vi "Test Read-Write Control Text.vi"(8 "error in (no error)":errorcluster) -> (0 "error out":errorcluster, 3 "Pass?":bool)   [LabVIEW 2020]
uses:
  G-Unicode/Types/UTF-8 String/UTF-8 String.lvclass/UTF-8 String.ctl
  G-Unicode/Dialog & User Interface/Polymorphic VIs/Write Control Text/Write Listbox Header (UTF-8 String).vi
  G-Unicode/Dialog & User Interface/Polymorphic VIs/Read Control Text/Read Listbox Header (UTF-8 String).vi
  47e1521e-4900-4e50-93d0-971907de44b7.vi
  G-Unicode/Dialog & User Interface/Polymorphic VIs/Write Control Text/Write Graph Plot Names (UTF-8 String).vi
  G-Unicode/Dialog & User Interface/Polymorphic VIs/Write Control Text/Write Graph Cursor Names (UTF-8 String).vi
  G-Unicode/Dialog & User Interface/Polymorphic VIs/Write Control Text/Write Graph Axis Labels (UTF-8 String).vi
  G-Unicode/Dialog & User Interface/Polymorphic VIs/Write Control Text/Write Table Headers (UTF-8 String).vi
  G-Unicode/Dialog & User Interface/Polymorphic VIs/Read Control Text/Read Table Headers (UTF-8 String).vi
  cbd299b7-ed5c-44d8-98e3-4b07b256a3af.vi
  97e6e9dd-fb41-465e-8130-768105b8566a.vi
  G-Unicode/Dialog & User Interface/Polymorphic VIs/Write Control Text/Write Multicolumn Listbox Headers (UTF-8 String).vi
  G-Unicode/Dialog & User Interface/Polymorphic VIs/Read Control Text/Read Multicolumn Listbox Headers (UTF-8 String).vi
  2cb1db3a-9545-49da-8e46-b28431192bfb.vi
  d3ca7cbe-fe55-4c08-9226-8df1279bea32.vi
  G-Unicode/Dialog & User Interface/Polymorphic VIs/Write Control Text/Write Radio Button Text (UTF-8 String).vi
  G-Unicode/Dialog & User Interface/Polymorphic VIs/Read Control Text/Read Radio Button Text (UTF-8 String).vi
  c66c8a8e-6384-46dd-ad34-c6b36e981c5f.vi
  G-Unicode/Dialog & User Interface/Polymorphic VIs/Write Control Text/Write Tab Pages (UTF-8 String).vi
  G-Unicode/Dialog & User Interface/Polymorphic VIs/Read Control Text/Read Tab Pages (UTF-8 String).vi
  11ce0e2c-e1a8-46a3-af78-7df26efc8245.vi
  G-Unicode/Dialog & User Interface/Polymorphic VIs/Write Control Text/Write Listbox Items (UTF-8 String).vi
  G-Unicode/Dialog & User Interface/Polymorphic VIs/Read Control Text/Read Listbox Items (UTF-8 String).vi
  c5b5f753-7993-4590-ab7a-38cd070e680f.vi
  G-Unicode/Dialog & User Interface/Polymorphic VIs/Write Control Text/Write Table Value (UTF-8 String).vi
  G-Unicode/Dialog & User Interface/Polymorphic VIs/Read Control Text/Read Table Value (UTF-8 String).vi
  d87d6912-68ee-4c4f-8e1f-9eaf2c3e8737.vi
  G-Unicode/Dialog & User Interface/Polymorphic VIs/Write Control Text/Write Ring Strings (UTF-8 String).vi
  G-Unicode/Dialog & User Interface/Polymorphic VIs/Read Control Text/Read Ring Strings (UTF-8 String).vi
  b51df372-b908-46a9-9cd9-1bce9bcba761.vi
  3f50c59c-438d-4159-8265-e7e5e4819d1d.vi
  G-Unicode/Dialog & User Interface/Polymorphic VIs/Write Control Text/Write 2D String Array Value (UTF-8 String).vi
  G-Unicode/Dialog & User Interface/Polymorphic VIs/Read Control Text/Read 2D String Array Value (UTF-8 String).vi
  f481c7ac-37a4-4879-9d59-93dd94c77838.vi
  G-Unicode/Dialog & User Interface/Polymorphic VIs/Write Control Text/Write 1D String Array Value (UTF-8 String).vi
  G-Unicode/Dialog & User Interface/Polymorphic VIs/Read Control Text/Read 1D String Array Value (UTF-8 String).vi
  2abff34c-ba54-40bb-bfb0-e7a9eb1a66c8.vi
  G-Unicode/Dialog & User Interface/Polymorphic VIs/Write Control Text/Write String Value (UTF-8 String).vi
  G-Unicode/Dialog & User Interface/Polymorphic VIs/Read Control Text/Read String Value (UTF-8 String).vi
  b9bba32d-5ca2-4258-b841-0da24b58b874.vi
  G-Unicode/Dialog & User Interface/Polymorphic VIs/Write Control Text/Write Multicolumn Listbox Items (UTF-8 String).vi
  G-Unicode/Dialog & User Interface/Polymorphic VIs/Read Control Text/Read Multicolumn Listbox Items (UTF-8 String).vi
  4c20338b-6e60-4a75-91ad-9e96f58f92b0.vi
  G-Unicode/Dialog & User Interface/Polymorphic VIs/Write Control Text/Write Listbox Header (UTF-8 String).vi/5206cb6b-04fb-41f5-a37e-29c14f142303.vi
  G-Unicode/Dialog & User Interface/Polymorphic VIs/Read Control Text/Read Listbox Header (UTF-8 String).vi/bfba3187-b22e-4285-8cc2-1816a803f974.vi
  47e1521e-4900-4e50-93d0-971907de44b7.vi/3a31b270-3bb6-4c58-a256-c5fcc2c98f09.vi
  47e1521e-4900-4e50-93d0-971907de44b7.vi/0ec5df2d-ef9b-4f84-a6a8-ffcedd45c4dc.vi
  G-Unicode/Dialog & User Interface/Polymorphic VIs/Write Control Text/Write Graph Plot Names (UTF-8 String).vi/5206cb6b-04fb-41f5-a37e-29c14f142303.vi
  G-Unicode/Dialog & User Interface/Polymorphic VIs/Write Control Text/Write Graph Cursor Names (UTF-8 String).vi/5206cb6b-04fb-41f5-a37e-29c14f142303.vi
  G-Unicode/Dialog & User Interface/Polymorphic VIs/Write Control Text/Write Graph Axis Labels (UTF-8 String).vi/5206cb6b-04fb-41f5-a37e-29c14f142303.vi
  G-Unicode/Dialog & User Interface/Polymorphic VIs/Write Control Text/Write Graph Axis Labels (UTF-8 String).vi/dd8e371b-806c-4d03-8f90-d02a4c0388fb.vi
  G-Unicode/Dialog & User Interface/Polymorphic VIs/Write Control Text/Write Table Headers (UTF-8 String).vi/5206cb6b-04fb-41f5-a37e-29c14f142303.vi
  G-Unicode/Dialog & User Interface/Polymorphic VIs/Write Control Text/Write Table Headers (UTF-8 String).vi/ac01c1c3-6448-4046-bb74-48d1977bc508.vi
  G-Unicode/Dialog & User Interface/Polymorphic VIs/Read Control Text/Read Table Headers (UTF-8 String).vi/eedf47bc-7647-4a54-abe9-23d54898c809.vi
  G-Unicode/Dialog & User Interface/Polymorphic VIs/Read Control Text/Read Table Headers (UTF-8 String).vi/0d5c28b1-d47f-4710-9fb4-2778fb7e7b81.vi
  cbd299b7-ed5c-44d8-98e3-4b07b256a3af.vi/3a31b270-3bb6-4c58-a256-c5fcc2c98f09.vi
  cbd299b7-ed5c-44d8-98e3-4b07b256a3af.vi/0ec5df2d-ef9b-4f84-a6a8-ffcedd45c4dc.vi
  97e6e9dd-fb41-465e-8130-768105b8566a.vi/3a31b270-3bb6-4c58-a256-c5fcc2c98f09.vi
  97e6e9dd-fb41-465e-8130-768105b8566a.vi/0ec5df2d-ef9b-4f84-a6a8-ffcedd45c4dc.vi
  G-Unicode/Dialog & User Interface/Polymorphic VIs/Write Control Text/Write Multicolumn Listbox Headers (UTF-8 String).vi/5206cb6b-04fb-41f5-a37e-29c14f142303.vi
  G-Unicode/Dialog & User Interface/Polymorphic VIs/Write Control Text/Write Multicolumn Listbox Headers (UTF-8 String).vi/ac01c1c3-6448-4046-bb74-48d1977bc508.vi
  G-Unicode/Dialog & User Interface/Polymorphic VIs/Read Control Text/Read Multicolumn Listbox Headers (UTF-8 String).vi/f6f7f231-7ddf-476b-a943-0386d848a5c9.vi
  G-Unicode/Dialog & User Interface/Polymorphic VIs/Read Control Text/Read Multicolumn Listbox Headers (UTF-8 String).vi/fba5a6d2-cdfe-4afc-9e2c-d2641906be0d.vi
  2cb1db3a-9545-49da-8e46-b28431192bfb.vi/3a31b270-3bb6-4c58-a256-c5fcc2c98f09.vi
  2cb1db3a-9545-49da-8e46-b28431192bfb.vi/0ec5df2d-ef9b-4f84-a6a8-ffcedd45c4dc.vi
  d3ca7cbe-fe55-4c08-9226-8df1279bea32.vi/3a31b270-3bb6-4c58-a256-c5fcc2c98f09.vi
  d3ca7cbe-fe55-4c08-9226-8df1279bea32.vi/0ec5df2d-ef9b-4f84-a6a8-ffcedd45c4dc.vi
  G-Unicode/Dialog & User Interface/Polymorphic VIs/Write Control Text/Write Radio Button Text (UTF-8 String).vi/5206cb6b-04fb-41f5-a37e-29c14f142303.vi
  G-Unicode/Dialog & User Interface/Polymorphic VIs/Read Control Text/Read Radio Button Text (UTF-8 String).vi/f6f7f231-7ddf-476b-a943-0386d848a5c9.vi
  c66c8a8e-6384-46dd-ad34-c6b36e981c5f.vi/3a31b270-3bb6-4c58-a256-c5fcc2c98f09.vi
  c66c8a8e-6384-46dd-ad34-c6b36e981c5f.vi/0ec5df2d-ef9b-4f84-a6a8-ffcedd45c4dc.vi
  G-Unicode/Dialog & User Interface/Polymorphic VIs/Write Control Text/Write Tab Pages (UTF-8 String).vi/5206cb6b-04fb-41f5-a37e-29c14f142303.vi
  G-Unicode/Dialog & User Interface/Polymorphic VIs/Read Control Text/Read Tab Pages (UTF-8 String).vi/f6f7f231-7ddf-476b-a943-0386d848a5c9.vi
  11ce0e2c-e1a8-46a3-af78-7df26efc8245.vi/3a31b270-3bb6-4c58-a256-c5fcc2c98f09.vi
  11ce0e2c-e1a8-46a3-af78-7df26efc8245.vi/0ec5df2d-ef9b-4f84-a6a8-ffcedd45c4dc.vi
  G-Unicode/Dialog & User Interface/Polymorphic VIs/Write Control Text/Write Listbox Items (UTF-8 String).vi/5206cb6b-04fb-41f5-a37e-29c14f142303.vi
  G-Unicode/Dialog & User Interface/Polymorphic VIs/Read Control Text/Read Listbox Items (UTF-8 String).vi/f6f7f231-7ddf-476b-a943-0386d848a5c9.vi
  c5b5f753-7993-4590-ab7a-38cd070e680f.vi/3a31b270-3bb6-4c58-a256-c5fcc2c98f09.vi
  c5b5f753-7993-4590-ab7a-38cd070e680f.vi/0ec5df2d-ef9b-4f84-a6a8-ffcedd45c4dc.vi
  G-Unicode/Dialog & User Interface/Polymorphic VIs/Write Control Text/Write Table Value (UTF-8 String).vi/5206cb6b-04fb-41f5-a37e-29c14f142303.vi
  G-Unicode/Dialog & User Interface/Polymorphic VIs/Read Control Text/Read Table Value (UTF-8 String).vi/f6f7f231-7ddf-476b-a943-0386d848a5c9.vi
  d87d6912-68ee-4c4f-8e1f-9eaf2c3e8737.vi/3a31b270-3bb6-4c58-a256-c5fcc2c98f09.vi
  d87d6912-68ee-4c4f-8e1f-9eaf2c3e8737.vi/0ec5df2d-ef9b-4f84-a6a8-ffcedd45c4dc.vi
  G-Unicode/Dialog & User Interface/Polymorphic VIs/Write Control Text/Write Ring Strings (UTF-8 String).vi/5206cb6b-04fb-41f5-a37e-29c14f142303.vi
  G-Unicode/Dialog & User Interface/Polymorphic VIs/Read Control Text/Read Ring Strings (UTF-8 String).vi/f6f7f231-7ddf-476b-a943-0386d848a5c9.vi
  b51df372-b908-46a9-9cd9-1bce9bcba761.vi/3a31b270-3bb6-4c58-a256-c5fcc2c98f09.vi
  b51df372-b908-46a9-9cd9-1bce9bcba761.vi/0ec5df2d-ef9b-4f84-a6a8-ffcedd45c4dc.vi
  3f50c59c-438d-4159-8265-e7e5e4819d1d.vi/3a31b270-3bb6-4c58-a256-c5fcc2c98f09.vi
  3f50c59c-438d-4159-8265-e7e5e4819d1d.vi/0ec5df2d-ef9b-4f84-a6a8-ffcedd45c4dc.vi
  G-Unicode/Dialog & User Interface/Polymorphic VIs/Write Control Text/Write 2D String Array Value (UTF-8 String).vi/5206cb6b-04fb-41f5-a37e-29c14f142303.vi
  G-Unicode/Dialog & User Interface/Polymorphic VIs/Read Control Text/Read 2D String Array Value (UTF-8 String).vi/f6f7f231-7ddf-476b-a943-0386d848a5c9.vi
  f481c7ac-37a4-4879-9d59-93dd94c77838.vi/3a31b270-3bb6-4c58-a256-c5fcc2c98f09.vi
  f481c7ac-37a4-4879-9d59-93dd94c77838.vi/0ec5df2d-ef9b-4f84-a6a8-ffcedd45c4dc.vi
  G-Unicode/Dialog & User Interface/Polymorphic VIs/Write Control Text/Write 1D String Array Value (UTF-8 String).vi/5206cb6b-04fb-41f5-a37e-29c14f142303.vi
  G-Unicode/Dialog & User Interface/Polymorphic VIs/Read Control Text/Read 1D String Array Value (UTF-8 String).vi/f6f7f231-7ddf-476b-a943-0386d848a5c9.vi
  2abff34c-ba54-40bb-bfb0-e7a9eb1a66c8.vi/3a31b270-3bb6-4c58-a256-c5fcc2c98f09.vi
  2abff34c-ba54-40bb-bfb0-e7a9eb1a66c8.vi/0ec5df2d-ef9b-4f84-a6a8-ffcedd45c4dc.vi
  G-Unicode/Dialog & User Interface/Polymorphic VIs/Write Control Text/Write String Value (UTF-8 String).vi/5206cb6b-04fb-41f5-a37e-29c14f142303.vi
  G-Unicode/Dialog & User Interface/Polymorphic VIs/Read Control Text/Read String Value (UTF-8 String).vi/bfba3187-b22e-4285-8cc2-1816a803f974.vi
  b9bba32d-5ca2-4258-b841-0da24b58b874.vi/3a31b270-3bb6-4c58-a256-c5fcc2c98f09.vi
  b9bba32d-5ca2-4258-b841-0da24b58b874.vi/0ec5df2d-ef9b-4f84-a6a8-ffcedd45c4dc.vi
  G-Unicode/Dialog & User Interface/Polymorphic VIs/Write Control Text/Write Multicolumn Listbox Items (UTF-8 String).vi/5206cb6b-04fb-41f5-a37e-29c14f142303.vi
  G-Unicode/Dialog & User Interface/Polymorphic VIs/Read Control Text/Read Multicolumn Listbox Items (UTF-8 String).vi/f6f7f231-7ddf-476b-a943-0386d848a5c9.vi
  4c20338b-6e60-4a75-91ad-9e96f58f92b0.vi/3a31b270-3bb6-4c58-a256-c5fcc2c98f09.vi
  4c20338b-6e60-4a75-91ad-9e96f58f92b0.vi/0ec5df2d-ef9b-4f84-a6a8-ffcedd45c4dc.vi
  G-Unicode/Private/Conversion/Text as Encoded String.vi
  G-Unicode/Private/Conversion/Polymorphic VIs/Text as Encoded String (UTF-8 String).vi
  G-Unicode/Private/Conversion/Encoded UTF-8 String to Encoded UTF-16LE String.vi
  G-Unicode/Types/UTF-8 String/New UTF-8 String.vi
  G-Unicode/Types/UTF-8 String/Read Encoded UTF-8 String.vi
  G-Unicode/Unicode/Encode String.vi
  G-Unicode/Private/Conversion/Text to UTF-8.vi
  G-Unicode/Private/Conversion/Polymorphic VIs/Text to UTF-8 (LabVIEW String).vi
  G-Unicode/Unicode/SubVIs/UTF-16 Byte Swap.vi
  G-Unicode/Private/Conversion/UTF-8 to Text.vi
  G-Unicode/Private/Conversion/Polymorphic VIs/UTF-8 to Text (LabVIEW String).vi
  G-Unicode/Private/Conversion/Encoded UTF-16LE String to Encoded UTF-8 String.vi
  G-Unicode/Unicode/Prepend BOM.vi
  G-Unicode/Unicode/SubVIs/Byte Order Marks.vi
  G-Unicode/Unicode/Detect BOM.vi
  G-Unicode/Private/User Interface/Write String.vi
  G-Unicode/Private/User Interface/Read String.vi
  G-Unicode/Unicode/Detect String Encoding.vi
  G-Unicode/Private/User Interface/Write String Array (1D).vi
  G-Unicode/Private/User Interface/Read String Array (1D).vi
  G-Unicode/Private/User Interface/Write String Array (2D).vi
  G-Unicode/Private/User Interface/Read String Array (2D).vi
  G-Unicode/Private/User Interface/Write Ring Control.vi
  G-Unicode/Private/User Interface/Read Ring Control.vi
  G-Unicode/Private/User Interface/Write MultCol Listbox Data.vi
  G-Unicode/Private/User Interface/Read MultCol Listbox Data.vi
  G-Unicode/Private/User Interface/Write MultCol Listbox Headers.vi
  G-Unicode/Private/User Interface/Read MultCol Listbox Headers.vi
  G-Unicode/Private/User Interface/Write Listbox Data.vi
  G-Unicode/Private/User Interface/Read Listbox Data.vi
  G-Unicode/Private/User Interface/Write Listbox Header.vi
  G-Unicode/Private/User Interface/Read Listbox Header.vi
  G-Unicode/Private/User Interface/Write Table Data.vi
  G-Unicode/Private/User Interface/Read Table Data.vi
  G-Unicode/Private/User Interface/Write Table Headers.vi
  G-Unicode/Private/User Interface/Read Table Headers.vi
  G-Unicode/Private/User Interface/Write Tab Control.vi
  G-Unicode/Private/User Interface/Read Tab Control.vi
  G-Unicode/Private/User Interface/Write Radio Buttons.vi
  G-Unicode/Private/User Interface/Read Radio Button Text.vi
  G-Unicode/Private/User Interface/Write Graph-Chart Plot Names.vi
  G-Unicode/Private/User Interface/Write Graph-Chart Axis Labels.vi
  G-Unicode/Private/User Interface/Write Graph-Chart Cursor Names.vi
  G-Unicode/Types/UTF-8 String/UTF-8 String.lvclass
  G-Unicode/G-Unicode.lvlib
panel:
  out "Waveform Graph":dbl[](graph)
  out "Waveform Chart":dbl(graph)
  in  "Radio Buttons":T1(radio)
  in  "Tab Control":enum32{"Page 1", "Page 2", "Page 3", "Page 4"}(tab)
  in  "Multicolumn Listbox":i32(listbox)
  in  "Listbox":i32(listbox)
  in  "Table Control":string[][](table)
  in  "Menu Ring":u16(ring)
  in  "Text Ring":u16(ring)
  in  "String Array (2D)":string[][](array[string])
  in  "String Array (1D)":string[](array[string])
  in  "String":string
  # "Note the dropdowns for the ring controls aren't rendered correctly, but when selected it looks OK."
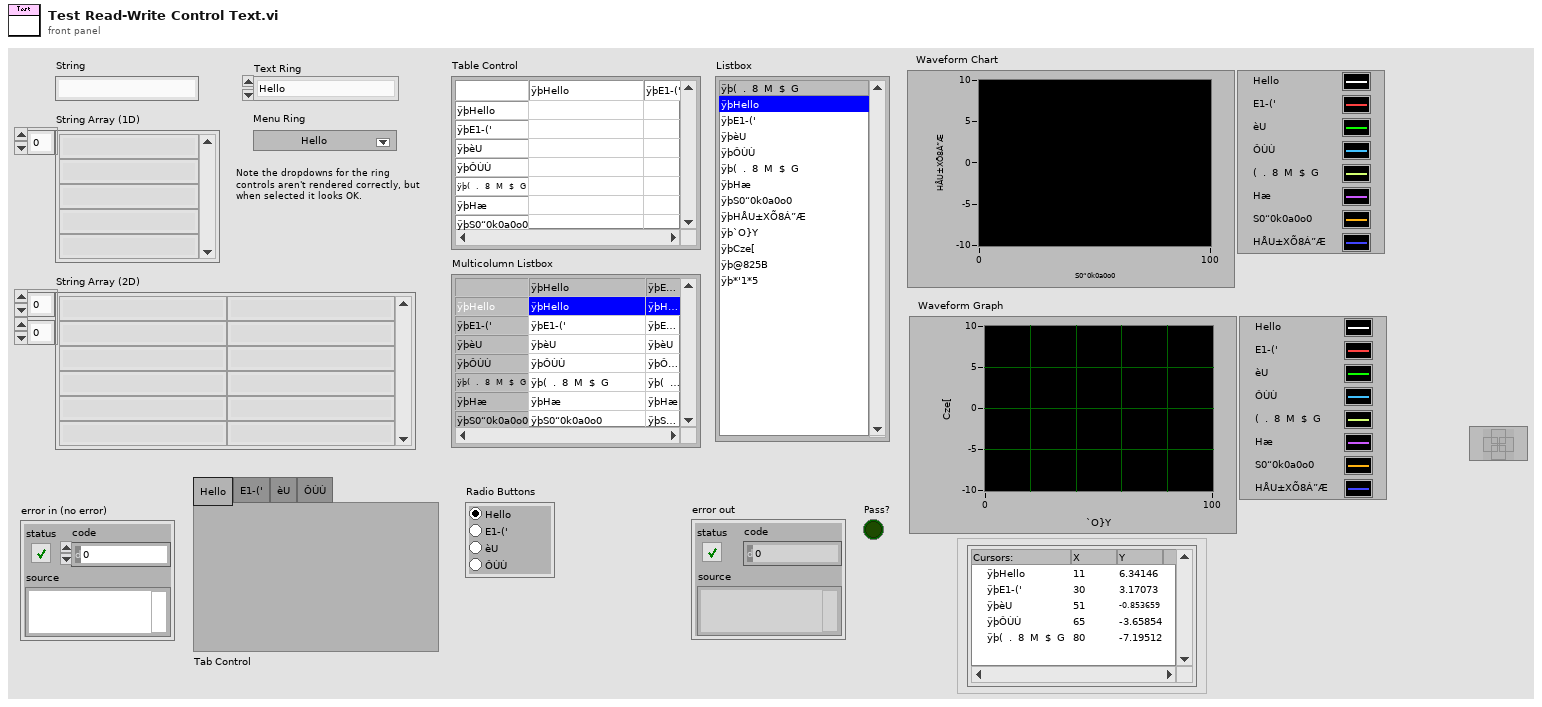
[diagram p1: front panel]
types:
  T1 = enum32{"Radio Selection 1", "Radio Selection 2", "Radio Selection 3", "Radio Selection 4"}
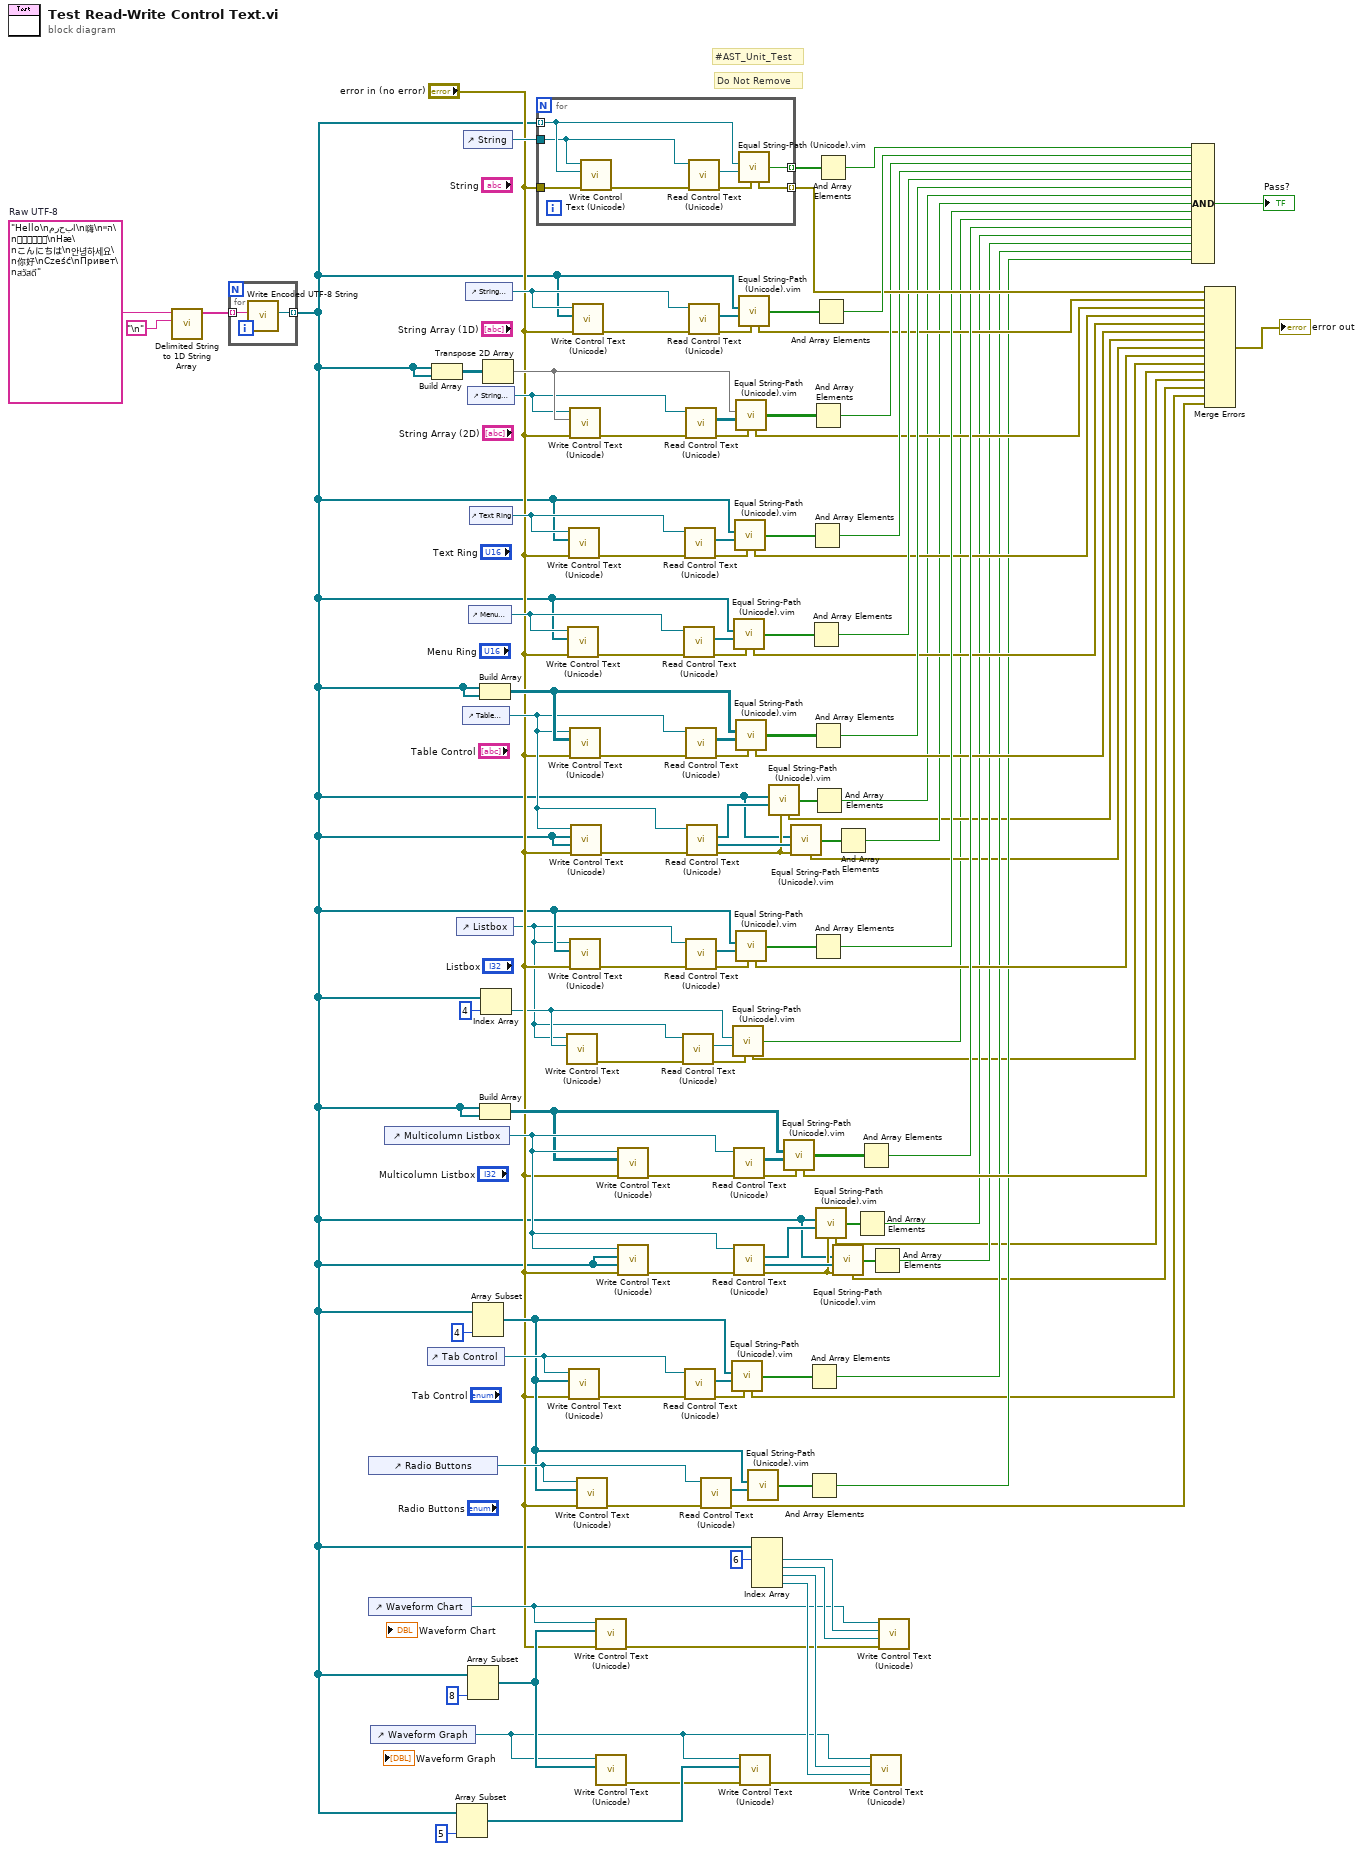
[diagram p0: block diagram]
diagram:
  w119 = "Hello\nمرحبا\n嗨\nהיי\nनमस्ते\nHæ\nこんにちは\n안녕하세요\n你好\nCześć\nПривет\nสวัสดี"  # Raw UTF-8
  # "Do Not Remove"
  # "#AST_Unit_Test"
  n1 = call <vilib>:"Delimited String to 1D String Array.vi"("delimiter"="\n", "delimited string"=w119) -> ("string array"=w118:string[])  [unwired: 9 in]
  n2 = for {
    tunnel: w118 -> [w122] mode=indexing
    tunnel: [w121] -> w6 mode=indexing
    n3 = call "Write Encoded UTF-8 String.vi"("Encoded UTF-8 String"=w122) -> ("UTF-8 String"=w121:refnum<class "UTF-8 String.lvclass">)  [unwired: 10 in]
  }
  n4 = control-ref of="Radio Buttons"() -> (w40:refnum<vi>)
  n5 = control-ref of="Waveform Chart"() -> (w48:refnum<vi>)
  n6 = control-ref of="Waveform Graph"() -> (w52:refnum<vi>)
  n7 = control-ref of="Multicolumn Listbox"() -> (w37:refnum<vi>)
  n8 = control-ref of="Tab Control"() -> (w43:refnum<vi>)
  n9 = Build Array(w6, w6) -> (w104:refnum<class "UTF-8 String.lvclass">[][])
  n10 = control-ref of="Listbox"() -> (w3:refnum<vi>)
  n11 = Array Subset(array=w6, length=5) -> (w60:refnum<class "UTF-8 String.lvclass">[])  [unwired: 1 in]
  n12 = control-ref of="Table Control"() -> (w22:refnum<vi>)
  n13 = control-ref of="String"() -> (w117:refnum<vi>)
  n14 = control-ref of="String Array (1D)"() -> (w47:refnum<vi>)
  n15 = control-ref of="String Array (2D)"() -> (w46:refnum<vi>)
  n16 = Array Subset(array=w6, length=8) -> (w58:refnum<class "UTF-8 String.lvclass">[])  [unwired: 1 in]
  n17 = control-ref of="Menu Ring"() -> (w44:refnum<vi>)
  n18 = control-ref of="Text Ring"() -> (w45:refnum<vi>)
  n19 = Array Subset(array=w6, length=4) -> (w39:refnum<class "UTF-8 String.lvclass">[])  [unwired: 1 in]
  n20 = Build Array(w6, w6) -> (w90:refnum<class "UTF-8 String.lvclass">[][])
  n21 = Build Array(w6, w6) -> (w36:refnum<class "UTF-8 String.lvclass">[][])
  n22 = Index Array(array=w6, index=4) -> (element=w4:refnum<class "UTF-8 String.lvclass">)
  n23 = Transpose 2D Array(2D array=w104) -> (transposed array=w102:refnum<class "UTF-8 String.lvclass">[][])
  n24 = for {
    tunnel: w117 -> [w123]
    tunnel: w6 -> [w125] mode=indexing
    tunnel: "error in (no error)" -> [w129]
    tunnel: [w126] -> w108 mode=indexing
    tunnel: [w128] -> w116 mode=indexing
    n25 = call-poly "Write Control Text (Unicode).vi"("error in"=w129, "Value"=w125, "Control Ref"=w123) -> ("error out"=w124:errorcluster)  [unwired: 8 in]
    n26 = call-poly "Read Control Text (Unicode).vi"("error in"=w124, "Control Ref"=w123) -> ("error out"=w127:errorcluster, "UTF-8 String"=w130:refnum<class "UTF-8 String.lvclass">)  [unwired: 8 in]
    n27 = call "Equal String-Path (Unicode).vim"("error in"=w127, "y"=w130, "x"=w125) -> ("error out"=w126:errorcluster, "Equal?"=w128:bool)  [unwired: 6 in]
  }
  n28 = call-poly "Write Control Text (Unicode).vi"("Value"=w4, "Control Ref"=w3) -> ("error out"=w9:errorcluster)  [unwired: 9 in]
  n29 = call-poly "Write Control Text (Unicode).vi"("error in"="error in (no error)", "Value"=w6, "Control Ref"=w44) -> ("error out"=w98:errorcluster)  [unwired: 8 in]
  n30 = call-poly "Write Control Text (Unicode).vi"("error in"="error in (no error)", "Value"=w6, "Control Ref"=w45) -> ("error out"=w99:errorcluster)  [unwired: 8 in]
  n31 = call-poly "Write Control Text (Unicode).vi"("error in"="error in (no error)", "Value"=w39, "Control Ref"=w43) -> ("error out"=w65:errorcluster)  [unwired: 8 in]
  n32 = call-poly "Write Control Text (Unicode).vi"("error in"="error in (no error)", "Value"=w102, "Control Ref"=w46) -> ("error out"=w106:errorcluster)  [unwired: 8 in]
  n33 = call-poly "Write Control Text (Unicode).vi"("error in"="error in (no error)", "Value"=w90, "Control Ref"=w22) -> ("error out"=w92:errorcluster)  [unwired: 8 in]
  n34 = call-poly "Write Control Text (Unicode).vi"("error in"="error in (no error)", "Value"=w6, "Control Ref"=w3) -> ("error out"=w86:errorcluster)  [unwired: 8 in]
  n35 = call-poly "Write Control Text (Unicode).vi"("error in"="error in (no error)", "Row Headers"=w6, "Column Headers"=w6, "Control Ref"=w22) -> ("error out"=w24:errorcluster)  [unwired: 7 in]
  n36 = call-poly "Write Control Text (Unicode).vi"("error in"="error in (no error)", "Value"=w6, "Control Ref"=w47) -> ("error out"=w111:errorcluster)  [unwired: 8 in]
  n37 = call-poly "Write Control Text (Unicode).vi"("error in"="error in (no error)", "Value"=w39, "Control Ref"=w40) -> ("error out"=w41:errorcluster)  [unwired: 8 in]
  n38 = call-poly "Write Control Text (Unicode).vi"("error in"="error in (no error)", "Plot Names"=w58, "Control Ref"=w48) -> ("error out"=w49:errorcluster)  [unwired: 8 in]
  n39 = call-poly "Write Control Text (Unicode).vi"("Plot Names"=w58, "Control Ref"=w52) -> ("error out"=w51:errorcluster)  [unwired: 9 in]
  n40 = call-poly "Write Control Text (Unicode).vi"("error in"="error in (no error)", "Value"=w36, "Control Ref"=w37) -> ("error out"=w83:errorcluster)  [unwired: 8 in]
  n41 = call-poly "Write Control Text (Unicode).vi"("error in"="error in (no error)", "Row Headers"=w6, "Column Headers"=w6, "Control Ref"=w37) -> ("error out"=w33:errorcluster)  [unwired: 7 in]
  n42 = call-poly "Read Control Text (Unicode).vi"("error in"=w9, "Control Ref"=w3) -> ("error out"=w8:errorcluster, "Value"=w7:refnum<class "UTF-8 String.lvclass">)  [unwired: 8 in]
  n43 = call-poly "Read Control Text (Unicode).vi"("error in"=w98, "Control Ref"=w44) -> ("error out"=w72:errorcluster, "Value"=w97:refnum<class "UTF-8 String.lvclass">[])  [unwired: 8 in]
  n44 = call-poly "Read Control Text (Unicode).vi"("error in"=w99, "Control Ref"=w45) -> ("error out"=w74:errorcluster, "Value"=w100:refnum<class "UTF-8 String.lvclass">[])  [unwired: 8 in]
  n45 = call-poly "Read Control Text (Unicode).vi"("error in"=w65, "Control Ref"=w43) -> ("error out"=w63:errorcluster, "Value"=w64:refnum<class "UTF-8 String.lvclass">[])  [unwired: 8 in]
  n46 = call-poly "Read Control Text (Unicode).vi"("error in"=w106, "Control Ref"=w46) -> ("error out"=w76:errorcluster, "Value"=w105:refnum<class "UTF-8 String.lvclass">[][])  [unwired: 8 in]
  n47 = call-poly "Read Control Text (Unicode).vi"("error in"=w92, "Control Ref"=w22) -> ("error out"=w70:errorcluster, "Value"=w93:refnum<class "UTF-8 String.lvclass">[][])  [unwired: 8 in]
  n48 = call-poly "Read Control Text (Unicode).vi"("error in"=w86, "Control Ref"=w3) -> ("error out"=w68:errorcluster, "Value"=w87:refnum<class "UTF-8 String.lvclass">[])  [unwired: 8 in]
  n49 = call-poly "Read Control Text (Unicode).vi"("error in"=w24, "Control Ref"=w22) -> ("error out"=w12:errorcluster, "Row Headers"=w21:refnum<class "UTF-8 String.lvclass">[], "Column Headers"=w23:refnum<class "UTF-8 String.lvclass">[])  [unwired: 7 in]
  n50 = call-poly "Read Control Text (Unicode).vi"("error in"=w111, "Control Ref"=w47) -> ("error out"=w78:errorcluster, "Value"=w112:refnum<class "UTF-8 String.lvclass">[])  [unwired: 8 in]
  n51 = call-poly "Read Control Text (Unicode).vi"("error in"=w41, "Control Ref"=w40) -> ("error out"=w25:errorcluster, "Value"=w42:refnum<class "UTF-8 String.lvclass">[])  [unwired: 8 in]
  n52 = call "Equal String-Path (Unicode).vim"("error in"=w63, "y"=w64, "x"=w39) -> ("error out"=w26:errorcluster, "Equal?"=w62:bool[])  [unwired: 6 in]
  n53 = call "Equal String-Path (Unicode).vim"("error in"=w8, "y"=w7, "x"=w4) -> ("error out"=w1:errorcluster, "Equal?"=w2:bool)  [unwired: 6 in]
  n54 = call "Equal String-Path (Unicode).vim"("error in"=w72, "y"=w97, "x"=w6) -> ("error out"=w71:errorcluster, "Equal?"=w96:bool[])  [unwired: 6 in]
  n55 = call-poly "Read Control Text (Unicode).vi"("error in"=w83, "Control Ref"=w37) -> ("error out"=w80:errorcluster, "Value"=w82:refnum<class "UTF-8 String.lvclass">[][])  [unwired: 8 in]
  n56 = call-poly "Read Control Text (Unicode).vi"("error in"=w33, "Control Ref"=w37) -> ("error out"=w15:errorcluster, "Row Headers"=w34:refnum<class "UTF-8 String.lvclass">[], "Column Headers"=w35:refnum<class "UTF-8 String.lvclass">[])  [unwired: 7 in]
  n57 = call "Equal String-Path (Unicode).vim"("error in"=w74, "y"=w100, "x"=w6) -> ("error out"=w73:errorcluster, "Equal?"=w101:bool[])  [unwired: 6 in]
  n58 = call "Equal String-Path (Unicode).vim"("error in"=w76, "y"=w105, "x"=w102) -> ("error out"=w75:errorcluster, "Equal?"=w107:bool[][])  [unwired: 6 in]
  n59 = call "Equal String-Path (Unicode).vim"("error in"=w70, "y"=w93, "x"=w90) -> ("error out"=w69:errorcluster, "Equal?"=w91:bool[][])  [unwired: 6 in]
  n60 = call "Equal String-Path (Unicode).vim"("error in"=w68, "y"=w87, "x"=w6) -> ("error out"=w67:errorcluster, "Equal?"=w88:bool[])  [unwired: 6 in]
  n61 = call "Equal String-Path (Unicode).vim"("error in"=w78, "y"=w112, "x"=w6) -> ("error out"=w77:errorcluster, "Equal?"=w110:bool[])  [unwired: 6 in]
  n62 = call-poly "Write Control Text (Unicode).vi"("error in"=w51, "Cursor Names"=w60, "Control Ref"=w52) -> ("error out"=w50:errorcluster)  [unwired: 8 in]
  n63 = call "Equal String-Path (Unicode).vim"("y"=w42, "x"=w39) -> ("Equal?"=w38:bool[])  [unwired: 7 in, 1 out]
  n64 = Index Array(array=w6, index #1=6 ("index")) -> (element #1=w56:refnum<class "UTF-8 String.lvclass">, element #2=w55:refnum<class "UTF-8 String.lvclass">, element #3=w54:refnum<class "UTF-8 String.lvclass">, element #4=w53:refnum<class "UTF-8 String.lvclass">)  [unwired: 3 in]
  n65 = call "Equal String-Path (Unicode).vim"("error in"=w12, "y"=w23, "x"=w6) -> ("error out"=w10:errorcluster, "Equal?"=w20:bool[])  [unwired: 6 in]
  n66 = call "Equal String-Path (Unicode).vim"("error in"=w80, "y"=w82, "x"=w36) -> ("error out"=w79:errorcluster, "Equal?"=w84:bool[][])  [unwired: 6 in]
  n67 = call "Equal String-Path (Unicode).vim"("error in"=w12, "y"=w21, "x"=w6) -> ("error out"=w11:errorcluster, "Equal?"=w19:bool[])  [unwired: 6 in]
  n68 = And Array Elements(Boolean array=w62) -> (logical AND=w29:bool)
  n69 = And Array Elements(Boolean array=w38) -> (logical AND=w30:bool)
  n70 = And Array Elements(Boolean array=w96) -> (logical AND=w94:bool)
  n71 = And Array Elements(Boolean array=w101) -> (logical AND=w95:bool)
  n72 = And Array Elements(Boolean array=w107) -> (logical AND=w103:bool)
  n73 = And Array Elements(Boolean array=w91) -> (logical AND=w89:bool)
  n74 = And Array Elements(Boolean array=w88) -> (logical AND=w85:bool)
  n75 = And Array Elements(Boolean array=w20) -> (logical AND=w18:bool)
  n76 = And Array Elements(Boolean array=w110) -> (logical AND=w109:bool)
  n77 = call "Equal String-Path (Unicode).vim"("error in"=w15, "y"=w35, "x"=w6) -> ("error out"=w13:errorcluster, "Equal?"=w32:bool[])  [unwired: 6 in]
  n78 = And Array Elements(Boolean array=w116) -> (logical AND=w115:bool)
  n79 = call "Equal String-Path (Unicode).vim"("error in"=w15, "y"=w34, "x"=w6) -> ("error out"=w14:errorcluster, "Equal?"=w31:bool[])  [unwired: 6 in]
  n80 = And Array Elements(Boolean array=w19) -> (logical AND=w17:bool)
  n81 = And Array Elements(Boolean array=w32) -> (logical AND=w28:bool)
  n82 = And Array Elements(Boolean array=w84) -> (logical AND=w81:bool)
  n83 = call-poly "Write Control Text (Unicode).vi"("error in"=w50, "Y Axis"=w53, "X Axis"=w54, "Control Ref"=w52) -> ()  [unwired: 7 in, 1 out]
  n84 = And Array Elements(Boolean array=w31) -> (logical AND=w27:bool)
  n85 = call-poly "Write Control Text (Unicode).vi"("error in"=w49, "Y Axis"=w55, "X Axis"=w56, "Control Ref"=w48) -> ()  [unwired: 7 in, 1 out]
  n86 = Compound Arithmetic op=AND(w115, w109, w103, w95, w94, w89, w18, w17, w85, w2, w81, w28, w27, w29, w30) -> (→"Pass?":bool)
  n87 = Merge Errors(w108, w77, w75, w73, w71, w69, w10, w11, w67, w1, w79, w13, w14, w26, w25) -> (→"error out":errorcluster)
